vi "Check_posn_tl.vi"(5 "error in (no error)":errorcluster, 6 "Channel Name":string, 7 "Valve Number":i32 max=9 step=1, 8 "Port Name":string) -> (0 "error out":errorcluster, 1 "Position":i32, 3 "Valve Number":i32)   [LabVIEW 2010]
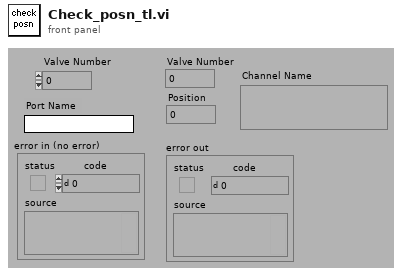
[diagram p1: front panel]
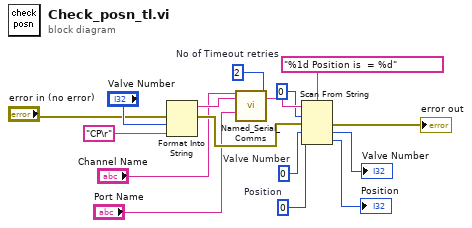
[diagram p0: block diagram]
diagram:
  w2 = 2  # No of Timeout retries
  w4 = 0  # Position
  w5 = 0  # Valve Number
  n1 = Format Into String(error in="error in (no error)", "Valve Number", "CP\r") -> (resulting string=w14:string, error out=w6:errorcluster)  [unwired: 2 in]
  n2 = call "Named_Serial_Comms.vi"("Channel Name"="Channel Name", "Write String"=w14, "!Timeout retries"=w2, "Port Name"="Port Name") -> ("Read"=w12:string)  [unwired: 5 in, 6 out]
  n3 = Scan From String(format string="%1d Position is  = %d", input string=w12, initial scan location=u32 0, error in=w6, default 1=w5, default 2=w4) -> (error out=→"error out":errorcluster, output 1=→"Valve Number":i32, output 2=→"Position":i32)  [unwired: 2 out]
